vi "Subvi counter to address.vi"(9 "Count":u16) -> (1 "Address":u32)   [LabVIEW 2017]
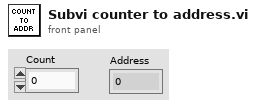
[diagram p1: front panel]
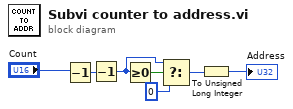
[diagram p0: block diagram]
diagram:
  n1 = Decrement(x="Count") -> (x-1=w7:u16)
  n2 = Decrement(x=w7) -> (x-1=w5:u16)
  n3 = Greater Or Equal To 0?(x=w5) -> (x >= 0?=w6:bool)
  n4 = Select(t=w5, s=w6, f=u16 0) -> (s? t:f=w2:u16)
  n5 = To Unsigned Long Integer(number=w2) -> (unsigned 32bit integer=→"Address":u32)
